vi "PID State Machine.vi"() -> ()   [LabVIEW 2021]
uses:
  Controls/Status Lights.ctl
  Controls/State Machine Data.ctl
  Controls/DAQ Refnums.ctl
  <vilib>/Utility/error.llb/Error Cluster From Error Code.vi
  <vilib>/ErrorRing/Error Ring.xnode
panel:
  in  "Manual Control Cluster":T1 {"Speed" scale=0.0..5.0}
  in  "Manual Control":bool
  in  "Simulated Pressure":dbl
  out "Speed":dbl
  out "Actuator Status":T2
  out "Pressure MPa":dbl
  in  "Target Pressure MPa":dbl
  out "Control State":string
  in  "Simulate":bool
  in  "Exit Button":bool
  in  "Start/Stop Controls":T3
  out "error out":errorcluster
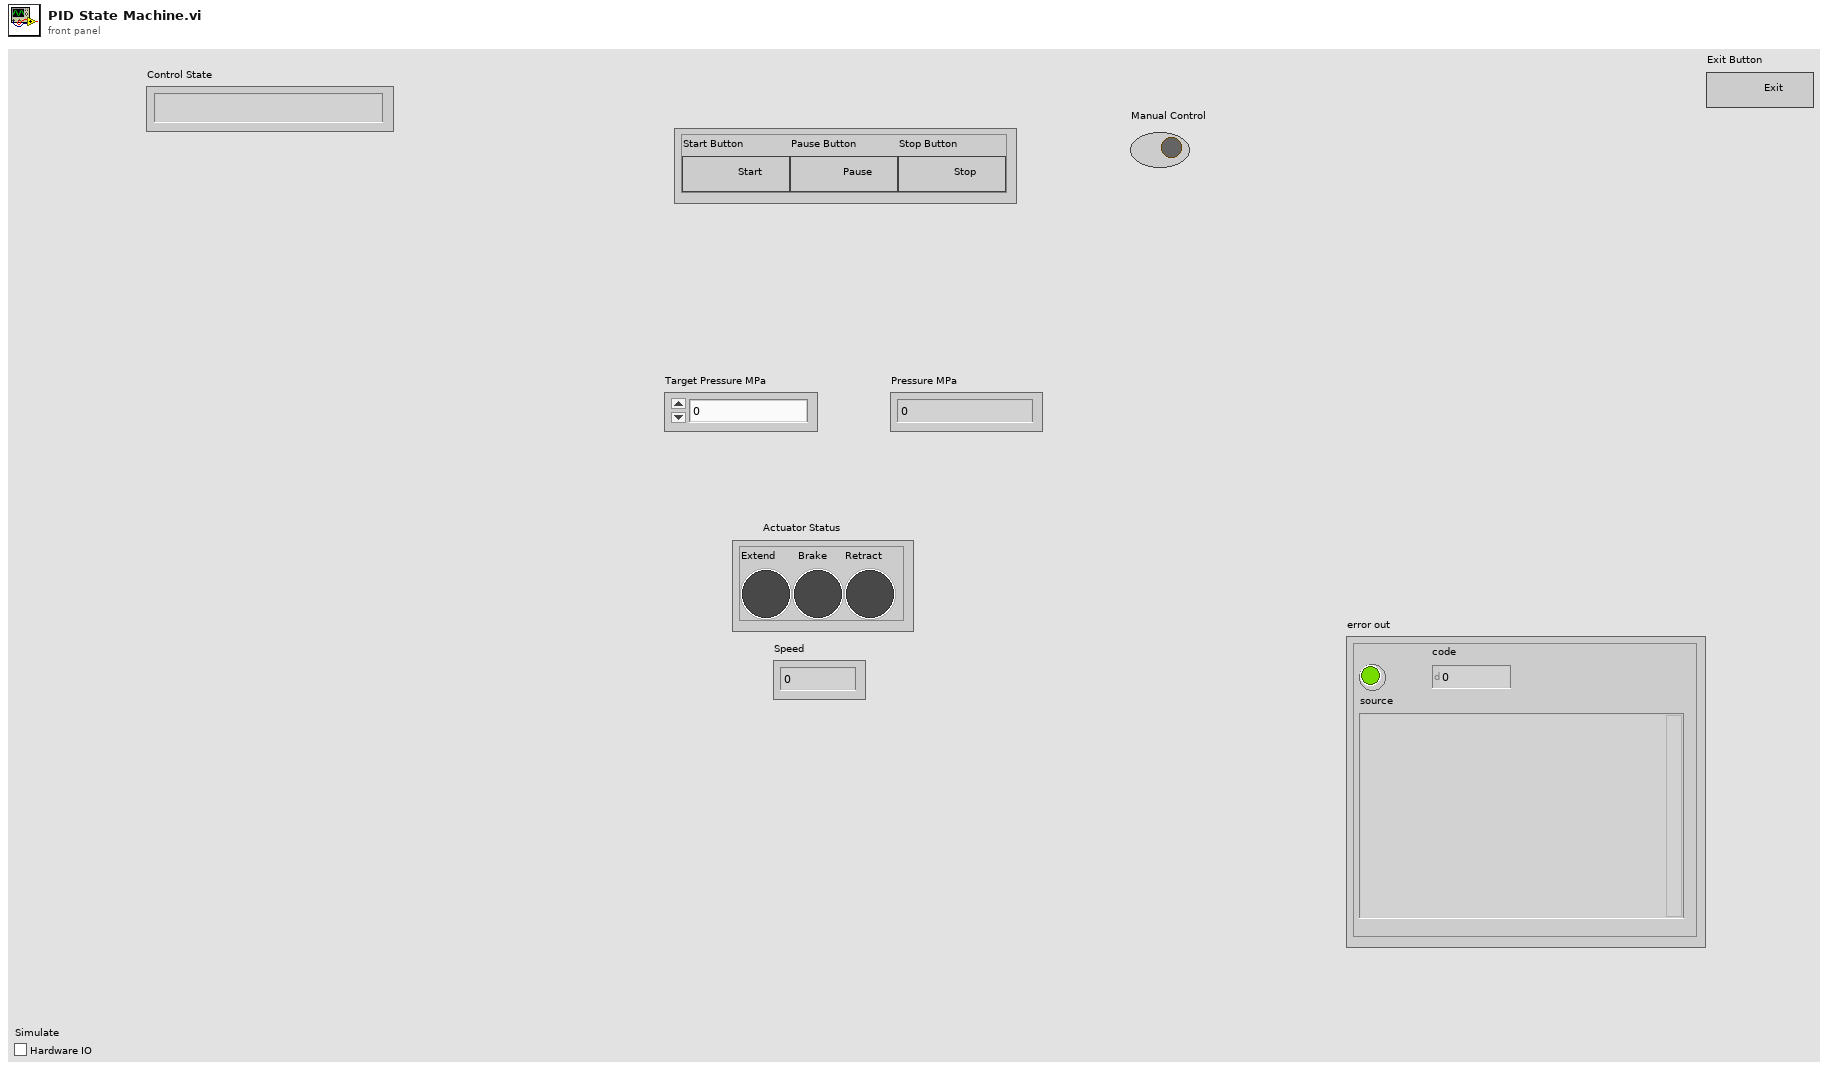
[diagram p1: front panel]
types:
  T1 = cluster{"Retract":bool, "Stop Button":bool, "Extend":bool, "Speed":dbl}
  T2 = typedef "Status Lights.ctl" = cluster{"Extend":bool, "Brake":bool, "Retract":bool}
  T3 = cluster{"Start Button":bool, "Pause Button":bool, "Stop Button":bool}
  T4 = cluster{"Start Button":refnum<vi>, "Pause Button":refnum<vi>, "Stop Button":refnum<vi>}
  T5 = typedef "State Machine Data.ctl" = cluster{"Control State":string, "Status Message":string, "Speed":dbl, "Pressure":dbl, "Target Pressure":dbl, "Apply Brake Ref":refnum<vi>, "Release Brake Ref":refnum<vi>, "Extend Ref":refnum<vi>, "Retract Ref":refnum<vi>, "Pressure Ref":refnum<vi>, "Data Display Ref":refnum<vi>, "Exit Button Ref":refnum<vi>, "Bool":bool, "Status":T2}
  T6 = typedef "DAQ Refnums.ctl" = cluster{"Direction Ref":refnum<k21>, "Brake Ref":refnum<k21>, "Speed Ref":refnum<k21>, "Pressure Ref":refnum<k21>}
  T7 = typedef "UI Data.ctl" = cluster{"Sampling State":string, "Status Message":string, "Speed":dbl, "Pressure":dbl, "Target Pressure":dbl, "Apply Brake Ref":refnum<vi>, "Release Brake Ref":refnum<vi>, "Extend Ref":refnum<vi>, "Retract Ref":refnum<vi>, "Pressure Ref":refnum<vi>, "Data Display Ref":refnum<vi>, "Exit Button Ref":refnum<vi>, "Speed Pressure Select":bool, "Status":T2}
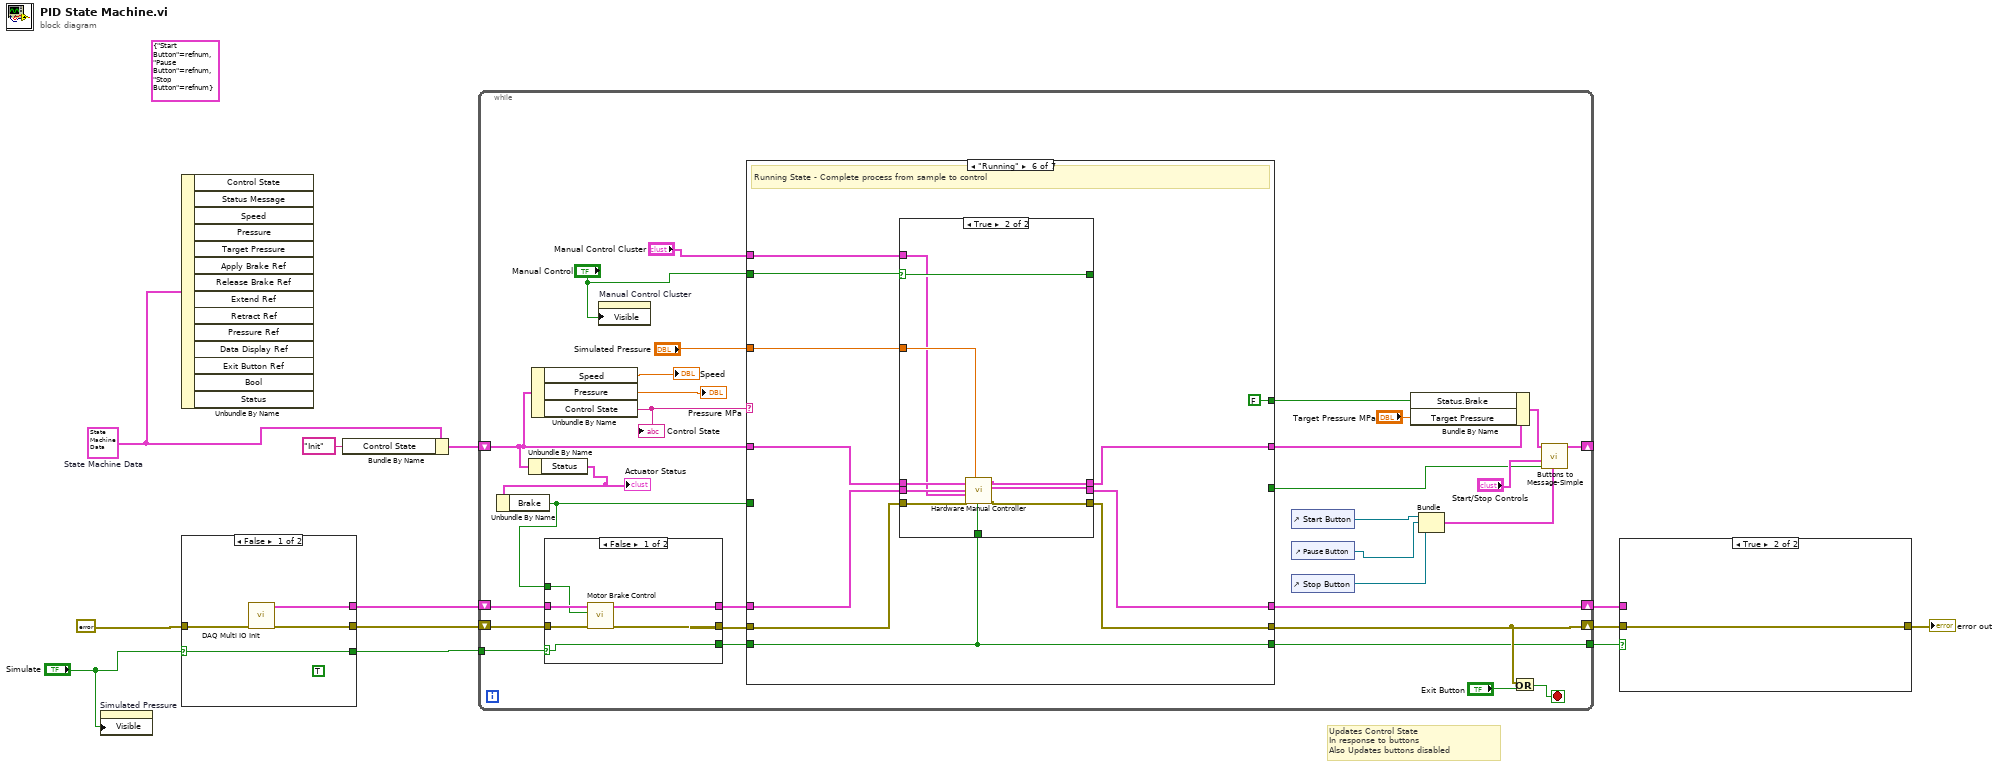
[diagram p0: block diagram]
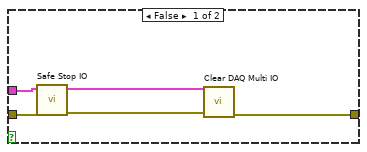
[diagram p2: hidden frame]
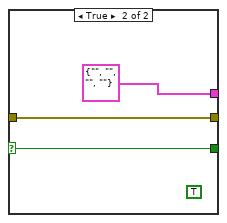
[diagram p3: hidden frame]
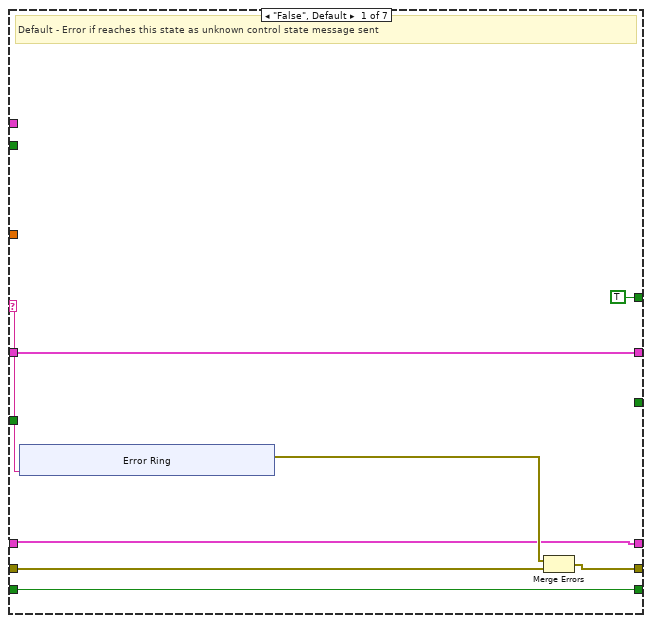
[diagram p5: hidden frame]
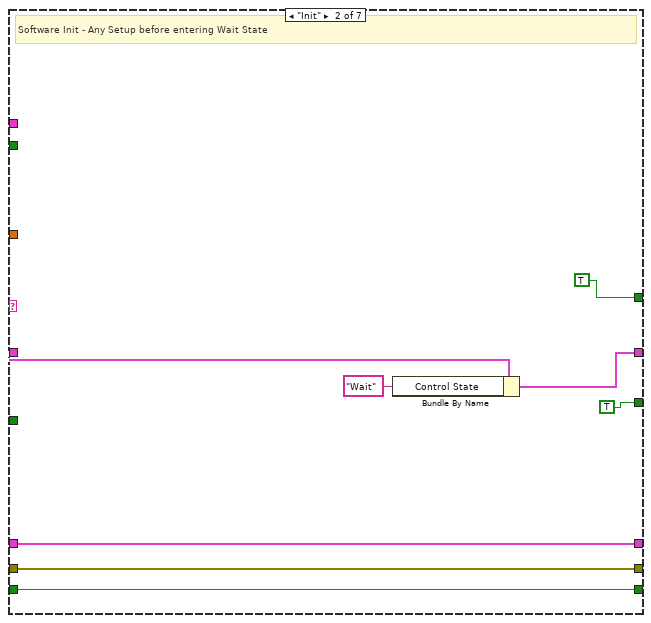
[diagram p6: hidden frame]
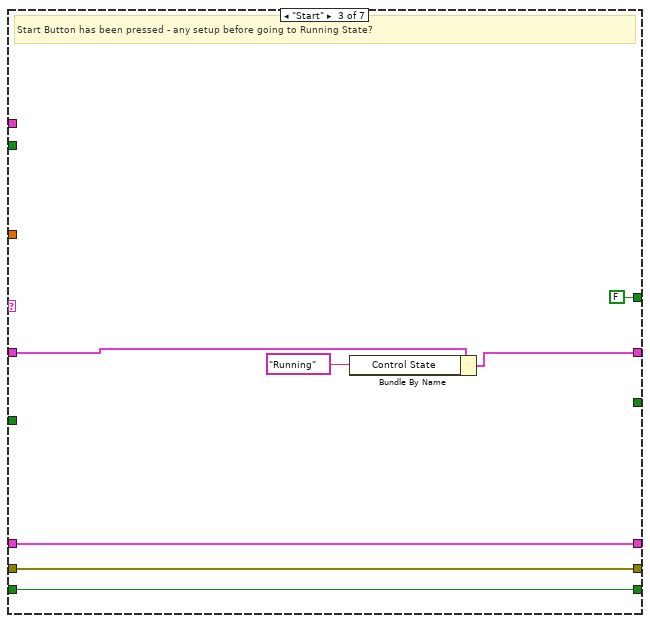
[diagram p7: hidden frame]
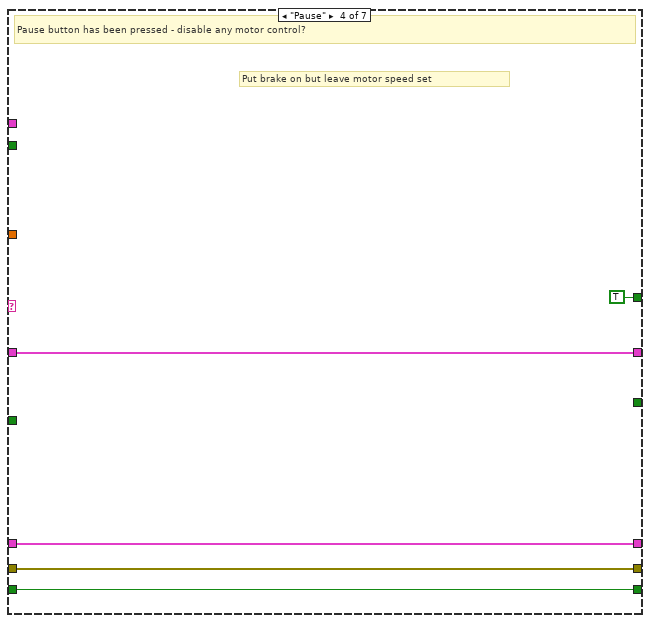
[diagram p8: hidden frame]
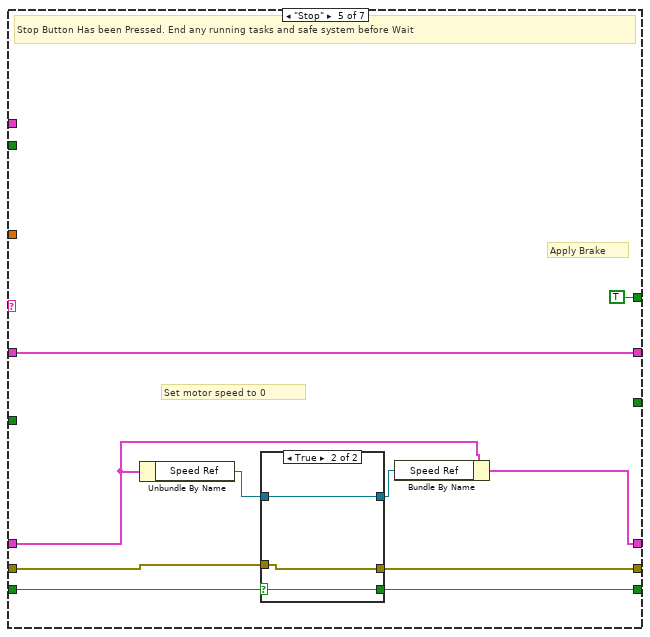
[diagram p9: hidden frame]
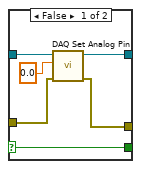
[diagram p10: hidden frame]
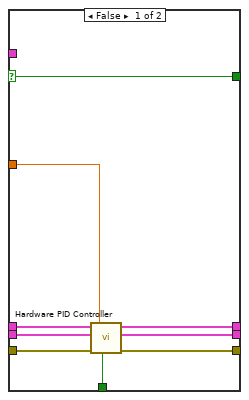
[diagram p11: hidden frame]
diagram:
  (unwired) T4 {"Start Button"=refnum, "Pause Button"=refnum, "Stop Button"=refnum}
  w12 = T5 {"Control State"="", "Status Message"="", "Speed"=0.0, "Pressure"=0.0, "Target Pressure"=0.0, "Apply Brake Ref"=refnum, "Release Brake Ref"=refnum, "Extend Ref"=refnum, "Retract Ref"=refnum, "Pressure Ref"=refnum, "Data Display Ref"=refnum, "Exit Button Ref"=refnum, "Bool"=TRUE, "Status"={"Extend"=FALSE, "Brake"=FALSE, "Retract"=FALSE}}  # State Machine Data
  # "Updates Control State\nIn response to buttons\nAlso Updates buttons disabled"
  n1 = property on="Simulated Pressure" class="DigNum (strict)"("Visible"="Simulate") -> ()  [unwired: 2 in, 2 out]
  n2 = Unbundle By Name(w12) -> ()  [unwired: 14 out]
  n3 = case shown="False" "Simulate" {
    selector: "Simulate" -> [w13 w17]
    tunnel: errorcluster {"status"=FALSE, "code"=0, "source"=""} ("error in") -> [w16 w18]
    tunnel: [w15 w18] -> w8
    tunnel: [w14 T6 {"Direction Ref"="", "Brake Ref"="", "Speed Ref"="", "Pressure Ref"=""} ("DAQ Ref Cluster")] -> w7
    tunnel: [w13 w17] -> w3
    frame False {
      (unwired) TRUE ("Visible")
      n4 = call "DAQ Multi IO Init.vi"("error in"=w16) -> ("error out"=w15:errorcluster, "DAQ Ref Cluster"=w14:T6)  [unwired: 9 in]
    }
    frame True {
      (unwired) TRUE ("Visible")
    }
  }
  n5 = Bundle By Name(cluster=w12, "Control State"="Init") -> (w11:T5)
  n6 = while {
    shift-right: [w47] -> _
    shift-left: w11 -> [w33]
    shift-right: [w41] -> w4
    shift-left: w8 -> [w31]
    shift-right: [w49] -> w5
    shift-left: w7 -> [w28]
    tunnel: w3 -> [w26]
    tunnel: [w24] -> w2
    stop <- w48 stop-if-true
    n7 = Unbundle By Name(w33) -> ("Status"=w32:T2)
    "Actuator Status" <- w32
    n8 = Unbundle By Name(w32) -> ("Brake"=w20:bool)
    n9 = Unbundle By Name(w33) -> ("Speed"=→"Speed":dbl, "Pressure"=→"Pressure MPa":dbl, "Control State"=w50:string)
    "Control State" <- w50
    n10 = case shown="False" w26 {
      selector: w26 -> [w51 w57]
      tunnel: w31 -> [w56 w58]
      tunnel: [w55 w59] -> w30
      tunnel: [w54 w58] -> w29
      tunnel: w28 -> [w53 w59]
      tunnel: w20 -> [w52 _]
      tunnel: [w51 w57] -> w25
      frame False {
        n11 = call "Motor Brake Control.vi"("error in (no error)"=w56, "Brake"=w52, "DAQ Ref Cluster in"=w53) -> ("error out"=w54:errorcluster, "DAQ Ref Cluster out"=w55:T6)  [unwired: 7 in]
      }
      frame True {
      }
    }
    n12 = property on="Manual Control Cluster" class="Clust"("Visible"="Manual Control") -> ()  [unwired: 2 in, 2 out]
    n13 = case shown="\"Running\"" w50 {
      selector: w50 -> [w62 _ _ _ _ _ _]
      tunnel: w33 -> [w64 w78 w86 w92 w104 w119 w146]
      tunnel: [w64 w79 w85 w92 w104 w120 w146] -> w38
      tunnel: [w67 w81 w88 w93 w98 w121 w147] -> w41
      tunnel: w29 -> [w65 w81 w88 w93 w97 w122 w147]
      tunnel: w30 -> [w63 w82 w89 w94 w100 w124 w148]
      tunnel: [w63 w82 w89 w94 w99 w123 w148] -> w49
      tunnel: [_ TRUE ("Reset") _ _ _ _ _] -> w39
      tunnel: [TRUE ("Brake") TRUE ("Status.Brake") FALSE ("Brake") TRUE ("Brake") TRUE ("Brake") FALSE ("Brake") w145] -> w34
      tunnel: w20 -> [_ _ _ _ _ _ w145]
      tunnel: w25 -> [w60 w75 w83 w90 w96 w117 w144]
      tunnel: [w60 w75 w83 w90 w95 w117 w144] -> w24
      tunnel: "Simulated Pressure" -> [_ _ _ _ _ w116 _]
      tunnel: "Manual Control" -> [_ _ _ _ _ w115 _]
      tunnel: "Manual Control Cluster" -> [_ _ _ _ _ w114 _]
      frame "False", Default {
        # "Default - Error if reaches this state as unknown control state message sent"
        n14 = xnode "Error Ring"("parameter 0"=w62) -> ("error out"=w66:errorcluster)
        n15 = Merge Errors(w66, w65) -> (w67:errorcluster)
      }
      frame "Init" {
        # "Software Init - Any Setup before entering Wait State"
        n16 = Bundle By Name(cluster=w78, "Control State"="Wait") -> (w79:T5)
      }
      frame "Start" {
        # "Start Button has been pressed - any setup before going to Running State?"
        n17 = Bundle By Name(cluster=w86, "Control State"="Running") -> (w85:T5)
      }
      frame "Pause" {
        # "Put brake on but leave motor speed set"
        # "Pause button has been pressed - disable any motor control?"
      }
      frame "Stop" {
        # "Apply Brake"
        # "Set motor speed to 0"
        # "Stop Button Has been Pressed. End any running tasks and safe system before Wait"
        n18 = Unbundle By Name(w100) -> ("Speed Ref"=w102:refnum<k21>)
        n19 = case shown="True" w96 {
          selector: w96 -> [w105 w111]
          tunnel: w102 -> [w110 w113]
          tunnel: [w109 w113] -> w101
          tunnel: [w108 w112] -> w98
          tunnel: w97 -> [w107 w112]
          tunnel: [w105 w111] -> w95
          frame False {
            n20 = call "DAQ Set Analog Pin.vi"("error in"=w107, "Voltage"=0.0, "task/channels in"=w110) -> ("error out"=w108:errorcluster, "task out"=w109:refnum<k21>)  [unwired: 6 in, 1 out]
          }
          frame True {
          }
        }
        n21 = Bundle By Name(cluster=w100, "Speed Ref"=w101) -> (w99:T6)
      }
      frame "Running" {
        # "Running State - Complete process from sample to control"
        n22 = case shown="True" w115 {
          selector: w115 -> [w125 w143]
          tunnel: w124 -> [w133 w139]
          tunnel: [w132 w137] -> w123
          tunnel: w122 -> [w131 w138]
          tunnel: [w130 w136] -> w121
          tunnel: [w129 w142] -> w120
          tunnel: w119 -> [w128 w141]
          tunnel: w117 -> [w127 w134]
          tunnel: w116 -> [w126 w140]
          tunnel: [w125 w143] -> _
          tunnel: w114 -> [_ w135]
          frame False {
            n23 = call "Hardware PID Controller.vi"("Simulate"=w127, "Simulated Actual Pressure"=w126, "error in (no error)"=w131, "DAQ Ref Cluster in"=w133, "State Machine Data"=w128) -> ("error out"=w130:errorcluster, "DAQ Ref Cluster out"=w132:T6, "Data Cluster out"=w129:T7)  [unwired: 4 in]
          }
          frame True {
            n24 = call "Hardware Manual Controller.vi"("Simulated"=w134, "Simulated Actual Pressure"=w140, "error in (no error)"=w138, "Manual Control Cluster"=w135, "DAQ Ref Cluster in"=w139, "State Machine Data"=w141) -> ("error out"=w136:errorcluster, "DAQ Ref Cluster out"=w137:T6, "Data Cluster out"=w142:T7)  [unwired: 3 in]
          }
        }
      }
      frame "Wait" {
        # "Wait State - Nothing active should be here"
      }
    }
    n25 = control-ref of="Start Button"() -> (w44:refnum<vi>)
    n26 = control-ref of="Pause Button"() -> (w45:refnum<vi>)
    n27 = control-ref of="Stop Button"() -> (w46:refnum<vi>)
    n28 = Bundle By Name(cluster=w38, "Status.Brake"=w34, "Target Pressure"="Target Pressure MPa") -> (w37:T5)
    n29 = Bundle("Start Button"=w44, "Pause Button"=w45, "Stop Button"=w46) -> (w42:T4)  [unwired: 1 in]
    n30 = Or(x=w41, y="Exit Button") -> (x .or. y?=w48:bool)
    n31 = call "Buttons to Message-Simple.vi"("Start/Stop Ref"=w42, "Reset"=w39, "Start/Stop Controls"="Start/Stop Controls", "State Machine Data"=w37) -> ("State Machine Data Out"=w47:T5)  [unwired: 7 in]
  }
  n32 = case shown="True" w2 {
    tunnel: [w153 w154] -> w6
    tunnel: w5 -> [w152 _]
    tunnel: w4 -> [w151 w154]
    frame False {
      n33 = call "Safe Stop IO.vi"("error in"=w151, "DAQ Ref Cluster"=w152) -> ("error out"=w149:errorcluster, "DAQ Ref Cluster Out"=w150:T6)  [unwired: 8 in]
      n34 = call "Clear DAQ Multi IO.vi"("error in"=w149, "DAQ Ref"=w150) -> ("error out"=w153:errorcluster)  [unwired: 9 in]
    }
    frame True {
    }
  }
  "error out" <- w6
